vi "set_ROIs_in_um.vi"(4 "error in (no error)":errorcluster, 5 "Value":T11, 6 "Container State":T10, 7 "Display State In":T1={"current frame index"=0, "number of images"=0, "ROI (frames)"={"ROI"=[]}, "control refs"={"frame"=refnum, "image"=refnum, "saveROIsButton"=refnum, "loadImageSwitch"=refnum, "loadROIsSwitch"=refnum, "saveROIsSwitch"=refnum, "loadImagePath"=refnum, "loadROIPath"=refnum, "redraw"=refnum}, "calibration"={"x"=0.0, "y"=0.0, "x unit"=enum."um", "y unit"=enum."um"}, "xpaths"={"x offset"="", "y offset"="", "z offset"=""}, "offset"=refnum, "XML description"="", "number of ROIs"=0.0, "ROI Tool Buttons Visible"={"Zoom Tool"=TRUE, "Selection Tool"=TRUE, "Pan Tool"=TRUE, "Point Tool"=TRUE, "Line Tool"=TRUE, "Rectangle Tool"=TRUE, "Rotated Rectangle Tool"=TRUE, "Polyline Tool"=TRUE, "Polygon Tool"=TRUE, "Freehand Tool"=TRUE, "Closed Freehand Tool"=TRUE, "Ellipse Tool"=TRUE, "Annulus Tool"=TRUE}, "ROI color"=6618880, "number color"=6618880, "enable ROI numbering?"=FALSE, "selected path to save ROIs"=path "", "starting path"=path "", "array of overlays"=[], "pointCollection"=refnum, "ROImode"=enum."IMAQROIs", "selected point ID"=0.0, "point radius"=5, "point colours"=[], "PlotAreaSize"={"Width"=0, "Height"=0}, "last action"=enum."not specified"} {"array of overlays"."overlay size" min=1}) -> (0 "error out":errorcluster, 3 "Display State Out":T1={"current frame index"=0, "number of images"=0, "ROI (frames)"={"ROI"=[]}, "control refs"={"frame"=refnum, "image"=refnum, "saveROIsButton"=refnum, "loadImageSwitch"=refnum, "loadROIsSwitch"=refnum, "saveROIsSwitch"=refnum, "loadImagePath"=refnum, "loadROIPath"=refnum, "redraw"=refnum}, "calibration"={"x"=0.0, "y"=0.0, "x unit"=enum."um", "y unit"=enum."um"}, "xpaths"={"x offset"="", "y offset"="", "z offset"=""}, "offset"=refnum, "XML description"="", "number of ROIs"=0.0, "ROI Tool Buttons Visible"={"Zoom Tool"=TRUE, "Selection Tool"=TRUE, "Pan Tool"=TRUE, "Point Tool"=TRUE, "Line Tool"=TRUE, "Rectangle Tool"=TRUE, "Rotated Rectangle Tool"=TRUE, "Polyline Tool"=TRUE, "Polygon Tool"=TRUE, "Freehand Tool"=TRUE, "Closed Freehand Tool"=TRUE, "Ellipse Tool"=TRUE, "Annulus Tool"=TRUE}, "ROI color"=6618880, "number color"=6618880, "enable ROI numbering?"=FALSE, "selected path to save ROIs"=path "", "starting path"=path "", "array of overlays"=[], "pointCollection"=refnum, "ROImode"=enum."IMAQROIs", "selected point ID"=0.0, "point radius"=5, "point colours"=[], "PlotAreaSize"={"Width"=0, "Height"=0}, "last action"=enum."not specified"} {"array of overlays"."overlay size" min=1})   [LabVIEW 2010, in "XImage.xctl"]
uses:
  XImage.xctl
  <vilib>/_xctls/Container State.ctl
  ROImicrons_frames_cluster.ctl
  ROImicrons_cluster.ctl
  state.ctl
  classes/SpaceVector/SpaceVector/SpaceVector.lvclass
  classes/PointCollection/PointCollection/PointCollection.lvclass
  ROI_frames_cluster.ctl
  control_refs_cluster.ctl
  calibration_cluster.ctl
  enumerations/unit.ctl
  xpath_cluster.ctl
  overlays_cluster.ctl
  ROI_mode_enum.ctl
  last_action_enum.ctl
  <vilib>/_xctls/XControlSupport.lvlib
  classes/Image/Image/Image.lvclass
panel:
  # "Replace the Value Control below with a Control of desired type.\nDo not remove this Control or the others from the connector pane.\nDo not change the connector pane pattern.\nThe Value control should always be the third terminal from top on the input side in the connector pane."
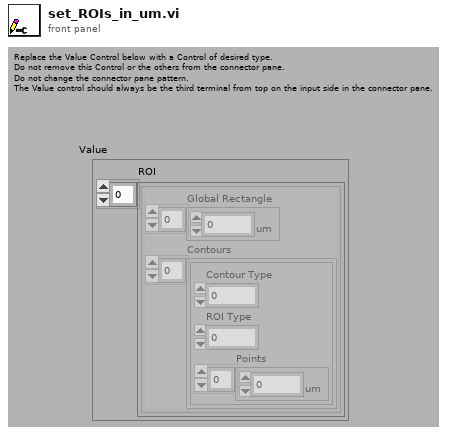
[diagram p1: front panel]
types:
  T1 = typedef "XImage.xctl/state.ctl" = cluster{"current frame index":i32, "number of images":i32, "ROI (frames)":T2, "control refs":T3, "calibration":T4, "xpaths":T6, "offset":refnum<class "SpaceVector.lvclass">, "XML description":string, "number of ROIs":dbl, "ROI Tool Buttons Visible":cluster{"Zoom Tool":bool, "Selection Tool":bool, "Pan Tool":bool, "Point Tool":bool, "Line Tool":bool, "Rectangle Tool":bool, "Rotated Rectangle Tool":bool, "Polyline Tool":bool, "Polygon Tool":bool, "Freehand Tool":bool, "Closed Freehand Tool":bool, "Ellipse Tool":bool, "Annulus Tool":bool}, "ROI color":u32, "number color":u32, "enable ROI numbering?":bool, "selected path to save ROIs":path, "starting path":path, "array of overlays":T7[], "pointCollection":refnum<class "PointCollection.lvclass">, "ROImode":T8, "selected point ID":dbl, "point radius":i32, "point colours":u32[], "PlotAreaSize":cluster{"Width":u32, "Height":u32}, "last action":T9}
  T2 = typedef "XImage.xctl/ROI_frames_cluster.ctl" = cluster{"ROI":cluster{"Global Rectangle":i32[], "Contours":cluster{"Contour Type":u32, "ROI Type":u32, "Points":i32[]}[]}[]}
  T3 = typedef "XImage.xctl/control_refs_cluster.ctl" = cluster{"frame":refnum<vi>, "image":refnum<vi>, "saveROIsButton":refnum<vi>, "loadImageSwitch":refnum<vi>, "loadROIsSwitch":refnum<vi>, "saveROIsSwitch":refnum<vi>, "loadImagePath":refnum<vi>, "loadROIPath":refnum<vi>, "redraw":refnum<vi>}
  T4 = typedef "XImage.xctl/calibration_cluster.ctl" = cluster{"x":dbl, "y":dbl, "x unit":T5, "y unit":T5}
  T5 = typedef "Image.lvclass/unit.ctl" = enum16{"um", "s"}
  T6 = typedef "XImage.xctl/xpath_cluster.ctl" = cluster{"x offset":string, "y offset":string, "z offset":string}
  T7 = typedef "XImage.xctl/overlays_cluster.ctl" = cluster{"overlay array":cluster{i32[][]}[], "overlay name":string, "color (red)":u32, "overlay size":i32, "overlay type":enum16{"crosshair", "circle"}}
  T8 = typedef "XImage.xctl/ROI_mode_enum.ctl" = enum16{"none", "IMAQROIs", "PointCollection"}
  T9 = typedef "XImage.xctl/last_action_enum.ctl" = enum16{"not specified", "image loaded", "frame changed", "ROIs changed"}
  T10 = typedef "XControlSupport.lvlib/Container State.ctl" = cluster{"Indicator?":bool, "Run Mode?":bool, " Refnum":refnum<vi>}
  T11 = typedef "XImage.xctl/ROImicrons_frames_cluster.ctl" = cluster{"ROI":T12[]}
  T12 = typedef "ROImicrons_cluster.ctl" = cluster{"Global Rectangle":dbl[unit][], "Contours":cluster{"Contour Type":u32, "ROI Type":u32, "Points":dbl[unit][]}[]}
  T13 = cluster{"Global Rectangle":i32[], "Contours":cluster{"Contour Type":u32, "ROI Type":u32, "Points":i32[]}[]}
  T14 = cluster{"Contour Type":u32, "ROI Type":u32, "Points":i32[]}
  T15 = cluster{"Global Rectangle":i32[], "Contours":cluster{"Contour Type":u32, "ROI Type":u32, "Points":i32[]}[]}[]
  T16 = cluster{"Contour Type":u32, "ROI Type":u32, "Points":dbl[unit][]}[]
  T17 = cluster{"[0]":dbl[unit], "[1]":dbl[unit], "[2]":dbl[unit], "[3]":dbl[unit]}
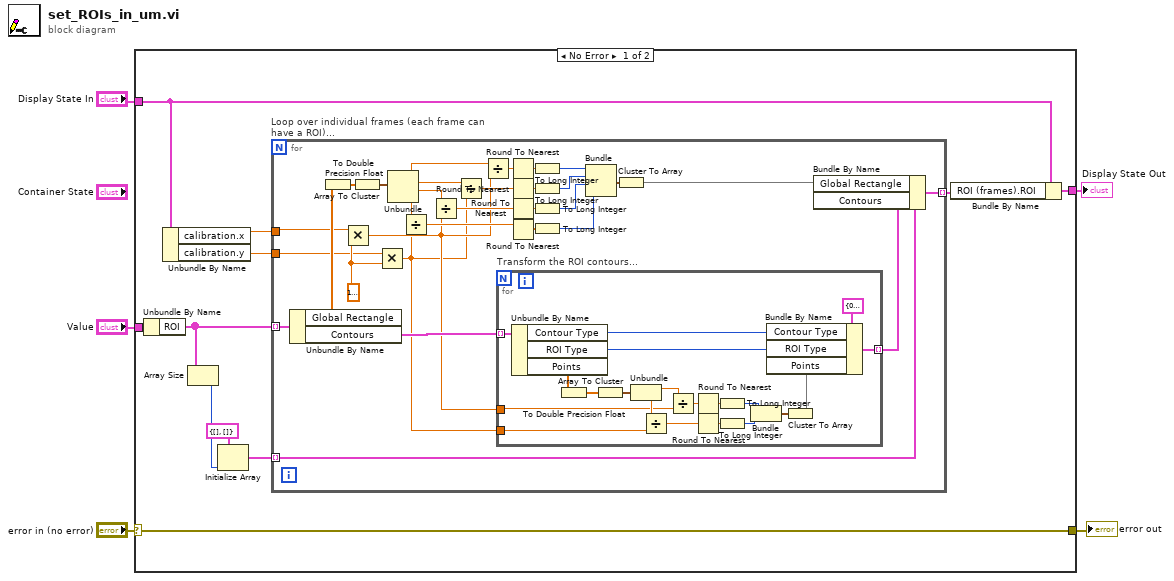
[diagram p0: block diagram]
diagram:
  n1 = case shown="No Error" "error in (no error)" {
    selector: "error in (no error)" -> [w6 w69]
    tunnel: "Display State In" -> [w16 w68]
    tunnel: [w15 w68] -> w4
    tunnel: "Value" -> [w14 _]
    tunnel: [w6 w69] -> w1
    frame No Error {
      n2 = Unbundle By Name(w14) -> ("ROI"=w10:T12[])
      n3 = Unbundle By Name(w16) -> ("calibration.x"=w13:dbl, "calibration.y"=w12:dbl)
      n4 = Array Size(array=w10) -> (size(s)=w9:i32)
      n5 = Initialize Array(T13 {"Global Rectangle"=[], "Contours"=[]} ("ROI"), w9) -> (w8:T15)
      n6 = for "Loop over individual frames (each frame can have a ROI)..." {
        tunnel: w10 -> [w47] mode=indexing
        tunnel: w13 -> [w39]
        tunnel: w12 -> [w37]
        tunnel: w8 -> [w21] mode=indexing
        tunnel: [w17] -> w7 mode=indexing
        w38 = dbl[unit] 1e-06 ("x*y")
        n7 = Unbundle By Name(w47) -> ("Global Rectangle"=w43:dbl[unit][], "Contours"=w24:T16)
        n8 = To Double Precision Float(number=w43) -> (double precision float=w44:dbl[unit][])
        n9 = Multiply(x=w39, y=w38) -> (x*y=w23:dbl[unit])
        n10 = Array To Cluster(array=w44) -> (cluster=w45:T17)
        n11 = Multiply(x=w37, y=w38) -> (x*y=w22:dbl[unit])
        n12 = Unbundle(w45) -> ("[0]"=w46:dbl[unit], "[1]"=w42:dbl[unit], "[2]"=w40:dbl[unit], "[3]"=w41:dbl[unit])
        n13 = Divide(x=w41, y=w22) -> (x/y=w25:dbl)
        n14 = Divide(x=w40, y=w23) -> (x/y=w26:dbl)
        n15 = Divide(x=w42, y=w22) -> (x/y=w30:dbl)
        n16 = Divide(x=w46, y=w23) -> (x/y=w36:dbl)
        n17 = for "Transform the ROI contours..." {
          tunnel: w24 -> [w67] mode=indexing
          tunnel: w23 -> [w52]
          tunnel: w22 -> [w51]
          tunnel: [w48] -> w20 mode=indexing
          n18 = Unbundle By Name(w67) -> ("Contour Type"=w65:u32, "ROI Type"=w64:u32, "Points"=w61:dbl[unit][])
          n19 = To Double Precision Float(number=w61) -> (double precision float=w63:dbl[unit][])
          n20 = Array To Cluster(array=w63) -> (cluster=w62:cluster{"[0]":dbl[unit], "[1]":dbl[unit]})
          n21 = Unbundle(w62) -> ("[0]"=w54:dbl[unit], "[1]"=w53:dbl[unit])
          n22 = Divide(x=w53, y=w51) -> (x/y=w59:dbl)
          n23 = Divide(x=w54, y=w52) -> (x/y=w55:dbl)
          n24 = Round To Nearest(number=w55) -> (nearest integer value=w56:dbl)
          n25 = Round To Nearest(number=w59) -> (nearest integer value=w58:dbl)
          n26 = To Long Integer(number=w56) -> (32bit integer=w57:i32)
          n27 = To Long Integer(number=w58) -> (32bit integer=w60:i32)
          n28 = Bundle(w57, w60) -> (w50:cluster{i32, i32})  [unwired: 1 in]
          n29 = Cluster To Array(cluster=w50) -> (array=w49:i32[])
          n30 = Bundle By Name(cluster=T14 {"Contour Type"=0, "ROI Type"=0, "Points"=[]}, "Contour Type"=w65, "ROI Type"=w64, "Points"=w49) -> (w48:T14)
        }
        n31 = Round To Nearest(number=w36) -> (nearest integer value=w35:dbl)
        n32 = Round To Nearest(number=w30) -> (nearest integer value=w33:dbl)
        n33 = Round To Nearest(number=w26) -> (nearest integer value=w32:dbl)
        n34 = Round To Nearest(number=w25) -> (nearest integer value=w31:dbl)
        n35 = To Long Integer(number=w35) -> (32bit integer=w34:i32)
        n36 = To Long Integer(number=w33) -> (32bit integer=w29:i32)
        n37 = To Long Integer(number=w32) -> (32bit integer=w28:i32)
        n38 = To Long Integer(number=w31) -> (32bit integer=w27:i32)
        n39 = Bundle(w34, w29, w28, w27) -> (w19:cluster{i32, i32, i32, i32})  [unwired: 1 in]
        n40 = Cluster To Array(cluster=w19) -> (array=w18:i32[])
        n41 = Bundle By Name(cluster=w21, "Global Rectangle"=w18, "Contours"=w20) -> (w17:T13)
      }
      n42 = Bundle By Name(cluster=w16, "ROI (frames).ROI"=w7) -> (w15:T1)
    }
    frame Error {
    }
  }
  "error out" <- w1
  "Display State Out" <- w4
